vi "HSV to RGB.vi"(8 "error in (no error)":errorcluster, 9 "Value(%)":dbl format="%#_13g", 10 "Saturation(%)":dbl format="%#_13g", 11 "Hue(°)":dbl format="%#_13g") -> (0 "error out":errorcluster, 1 "Blue":u8, 2 "Green":u8, 3 "Red":u8)   [LabVIEW 2018, in "Colour Lab.lvlib"]
uses:
  Colour Lab.lvlib
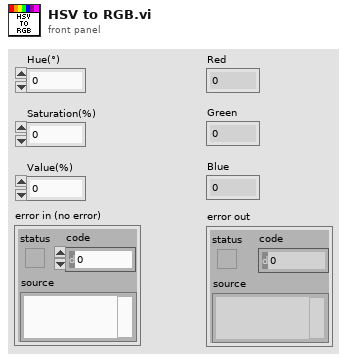
[diagram p1: front panel]
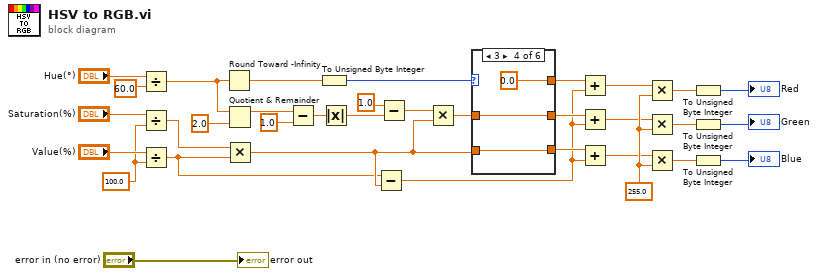
[diagram p0: block diagram]
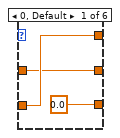
[diagram p2: hidden frame]
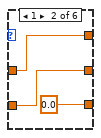
[diagram p3: hidden frame]
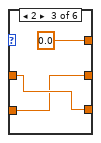
[diagram p4: hidden frame]
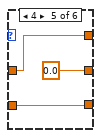
[diagram p5: hidden frame]
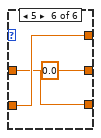
[diagram p6: hidden frame]
diagram:
  w1 = 100.0 ("y")
  w13 = 255.0 ("y")
  n1 = Divide(x="Hue(°)", y=60.0) -> (x/y=w23:dbl)
  n2 = Divide(x="Saturation(%)", y=w1) -> (x/y=w2:dbl)
  n3 = Divide(x="Value(%)", y=w1) -> (x/y=w4:dbl)
  n4 = Round Toward -Infinity(1:w23) -> (0:w22:dbl)
  n5 = Quotient & Remainder(x=w23, y=2.0) -> (x-y*floor(x/y)=w26:dbl)  [unwired: 1 out]
  n6 = Multiply(x=w2, y=w4) -> (x*y=w17:dbl)
  n7 = Subtract(x=w26, y=1.0) -> (x-y=w28:dbl)
  n8 = To Unsigned Byte Integer(number=w22) -> (unsigned 8bit integer=w18:u8)
  n9 = Absolute Value(x=w28) -> (abs(x)=w29:dbl)
  n10 = Subtract(x=w4, y=w17) -> (x-y=w8:dbl)
  n11 = Subtract(x=1.0, y=w29) -> (x-y=w31:dbl)
  n12 = Multiply(x=w31, y=w17) -> (x*y=w24:dbl)
  n13 = case shown="3" w18 {
    tunnel: w17 -> [w37 w39 w41 w45 w48 w52]
    tunnel: w24 -> [w36 w40 w42 w46 w49 w50]
    tunnel: [0.0 0.0 w42 w45 w48 w50] -> w9
    tunnel: [w36 w39 w41 w46 0.0 0.0] -> w10
    tunnel: [w37 w40 0.0 0.0 w49 w52] -> w11
    frame 0, Default {
    }
    frame 1 {
    }
    frame 2 {
    }
    frame 3 {
    }
    frame 4 {
    }
    frame 5 {
    }
  }
  n14 = Add(x=w11, y=w8) -> (x+y=w12:dbl)
  n15 = Add(x=w10, y=w8) -> (x+y=w6:dbl)
  n16 = Add(x=w9, y=w8) -> (x+y=w7:dbl)
  n17 = Multiply(x=w12, y=w13) -> (x*y=w16:dbl)
  n18 = Multiply(x=w6, y=w13) -> (x*y=w15:dbl)
  n19 = Multiply(x=w7, y=w13) -> (x*y=w14:dbl)
  n20 = To Unsigned Byte Integer(number=w16) -> (unsigned 8bit integer=→"Red":u8)
  n21 = To Unsigned Byte Integer(number=w15) -> (unsigned 8bit integer=→"Green":u8)
  n22 = To Unsigned Byte Integer(number=w14) -> (unsigned 8bit integer=→"Blue":u8)
  "error out" <- "error in (no error)"
